vi "hosts.deserialize.orderbook.commands.vi"(11 "DataIn":u64[](array[numeric])) -> (3 "OrderBook.Command[]":T1[](array[typedef]))   [LabVIEW 2020]
uses:
  arty/orderbook/orderbook.command.ctl
  arty/orderbook/orderbook.command.type.ctl
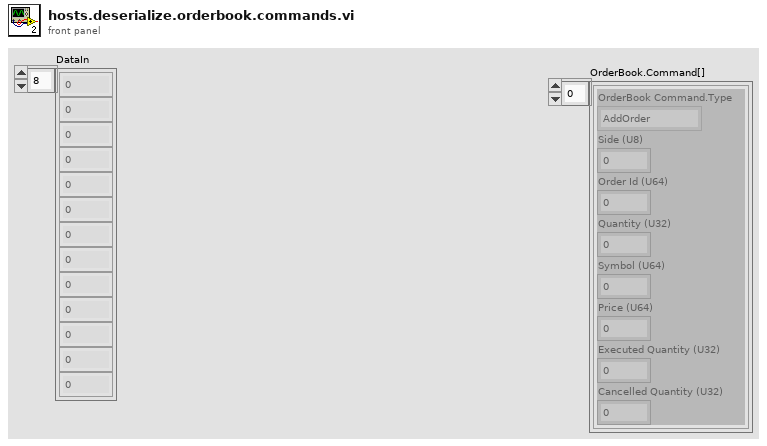
[diagram p1: front panel]
types:
  T1 = typedef "orderbook.command.ctl" = cluster{"OrderBook Command.Type":T2, "Side (U8)":u8, "Order Id (U64)":u64, "Quantity (U32)":u32, "Symbol (U64)":u64, "Price (U64)":u64, "Executed Quantity (U32)":u32, "Cancelled Quantity (U32)":u32}
  T2 = typedef "orderbook.command.type.ctl" = enum16{"AddOrder", "OrderExecuted", "ReduceSize", "ModifyOrder", "DeleteOrder", "Query"}
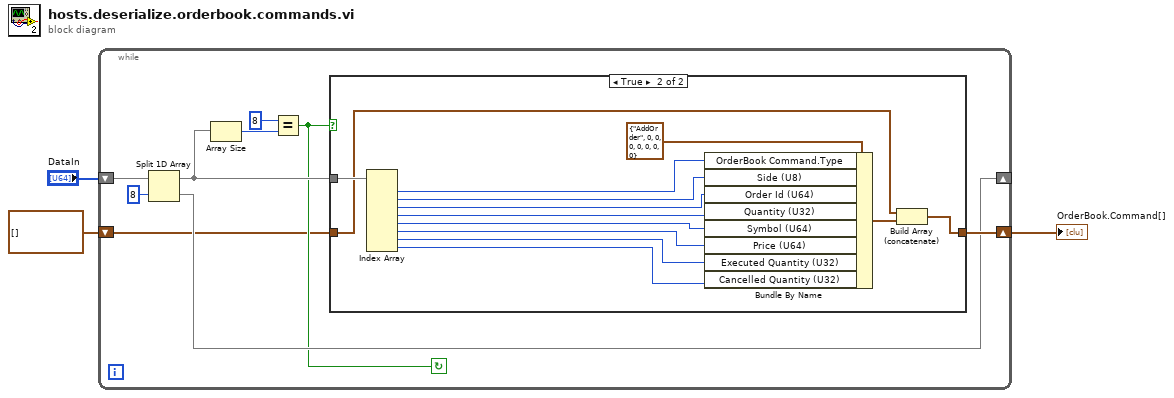
[diagram p0: block diagram]
diagram:
  n1 = while {
    shift-right: [w8] -> _
    shift-left: "DataIn" -> [w12]
    shift-right: [w10] -> w2
    shift-left: T1[] [] -> [w4]
    stop <- w5 continue-if-true
    n2 = Split 1D Array(array=w12, index=8) -> (first subarray=w9:u64[], second subarray=w8:u64[])
    n3 = Array Size(array=w9) -> (size(s)=w7:i32)
    n4 = Equal?(x=8, y=w7) -> (x = y?=w5:bool)
    n5 = case shown="True" w5 {
      tunnel: [w13 w15] -> w10
      tunnel: w9 -> [_ w17]
      tunnel: w4 -> [w13 w14]
      frame False {
      }
      frame True {
        n6 = Index Array(array=w17) -> (element #1=w25:u64, element #2=w24:u64, element #3=w23:u64, element #4=w22:u64, element #5=w21:u64, element #6=w20:u64, element #7=w19:u64, element #8=w18:u64)  [unwired: 8 in]
        n7 = Bundle By Name(cluster=T1 {"OrderBook Command.Type"=enum."AddOrder", "Side (U8)"=0, "Order Id (U64)"=0, "Quantity (U32)"=0, "Symbol (U64)"=0, "Price (U64)"=0, "Executed Quantity (U32)"=0, "Cancelled Quantity (U32)"=0} ("Cluster"), "OrderBook Command.Type"=w25, "Side (U8)"=w24, "Order Id (U64)"=w23, "Quantity (U32)"=w22, "Symbol (U64)"=w21, "Price (U64)"=w20, "Executed Quantity (U32)"=w19, "Cancelled Quantity (U32)"=w18) -> (w16:T1)
        n8 = Build Array (concatenate)(w14, w16) -> (w15:T1[])
      }
    }
  }
  "OrderBook.Command[]" <- w2
